vi "Destroy Message Enqueue References.vi"(8 "error in (no error)":errorcluster, 11 "Event-References":T1) -> (0 "error out":errorcluster)   [LabVIEW 2018, in "Actor.lvclass"]
uses:
  Actor.lvclass
  Message-Enqueue Refs.ctl
  Stop.ctl
  Launch.ctl
  Did Initialize.ctl
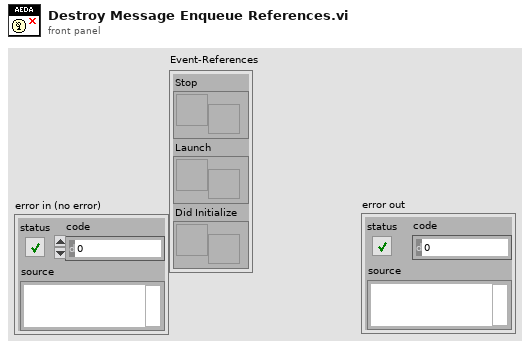
[diagram p1: front panel]
types:
  T1 = typedef "Actor.lvclass/Message-Enqueue Refs.ctl" = cluster{"Stop":refnum<user-event>, "Launch":refnum<user-event>, "Did Initialize":refnum<user-event>}
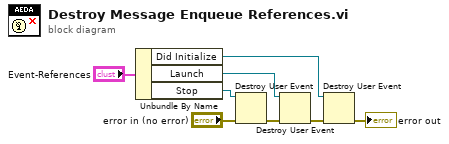
[diagram p0: block diagram]
diagram:
  n1 = Unbundle By Name("Event-References") -> ("Did Initialize"=w1:refnum<user-event>, "Launch"=w5:refnum<user-event>, "Stop"=w7:refnum<user-event>)
  n2 = Destroy User Event(user event=w7, error in="error in (no error)") -> (error out=w4:errorcluster)
  n3 = Destroy User Event(user event=w5, error in=w4) -> (error out=w3:errorcluster)
  n4 = Destroy User Event(user event=w1, error in=w3) -> (error out=→"error out":errorcluster)
